vi "Fractal.vi"() -> ()   [LabVIEW 2012]
uses:
  typedefs/t_LuaVIEW Reference.ctl
  subvis/private/LuaVIEW Pull (number).vi
  subvis/private/LuaVIEW Pull (U32).vi
  subvis/private/LuaVIEW Push (number).vi
panel:
  out "picture":picture
  # "This example uses a Lua-driven state machine to draw a fractal. Recursive and numerical algorithms\nare difficult to implement with elegance in LabVIEW, Lua by default has no support for graphics.\nTherefore the recursion and calculations are done with Lua, and the drawing with LabVIEW."
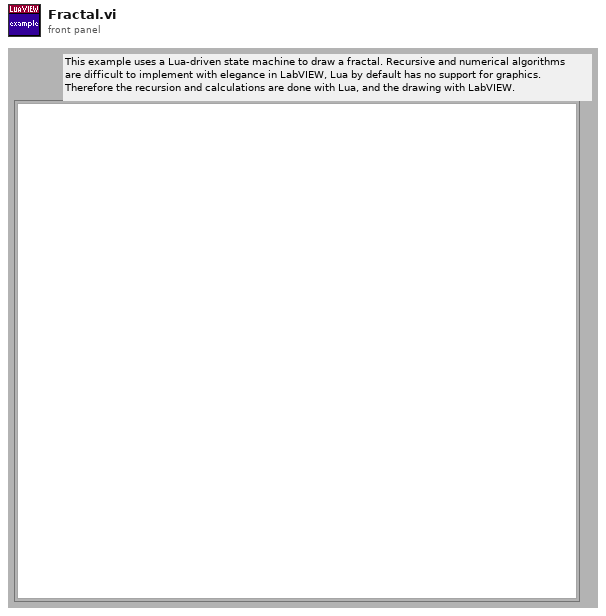
[diagram p1: front panel]
types:
  T1 = enum32{"execute", "initialize", "clear()", "line(num:x1,num:y1,num:x2,num:y2,U32:colour)", "num:width,num:height = dimensions()", "cleanup"}
  T2 = typedef "t_LuaVIEW Reference.ctl" = refnum<k1>
  T3 = typedef "LVBoundsTypeDef.ctl" = cluster{"Width":u32, "Height":u32}
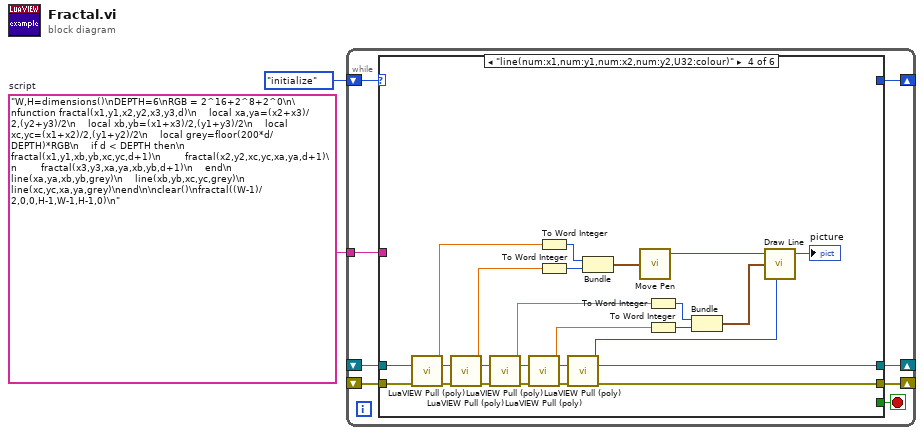
[diagram p0: block diagram]
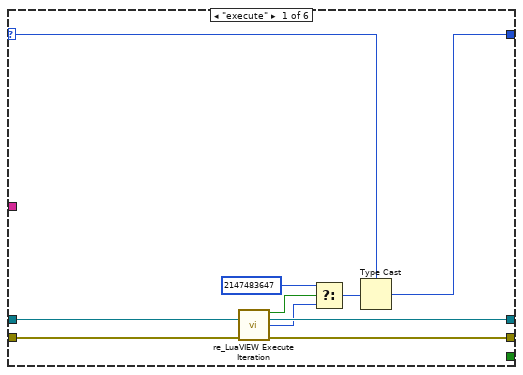
[diagram p2: hidden frame]
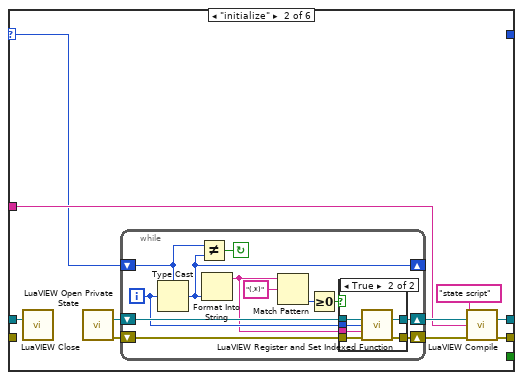
[diagram p3: hidden frame]
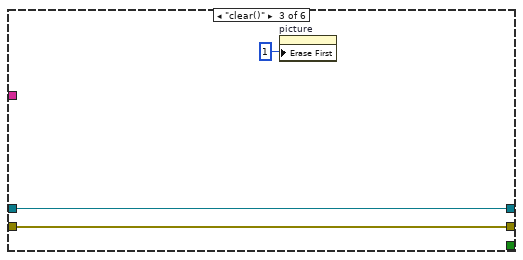
[diagram p5: hidden frame]
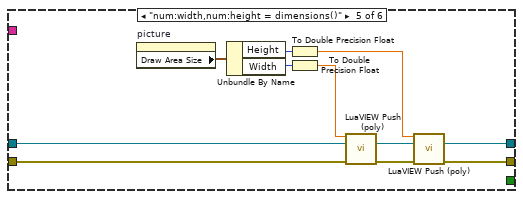
[diagram p6: hidden frame]
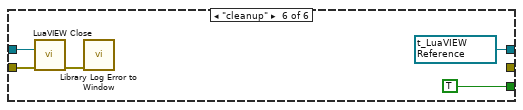
[diagram p7: hidden frame]
diagram:
  w1 = "W,H=dimensions()\nDEPTH=6\nRGB = 2^16+2^8+2^0\n\nfunction fractal(x1,y1,x2,y2,x3,y3,d)\n    local xa,ya=(x2+x3)/2,(y2+y3)/2\n    local xb,yb=(x1+x3)/2,(y1+y3)/2\n    local xc,yc=(x1+x2)/2,(y1+y2)/2\n    local grey=floor(200*d/DEPTH)*RGB\n    if d < DEPTH then\n        fractal(x1,y1,xb,yb,xc,yc,d+1)\n        fractal(x2,y2,xc,yc,xa,ya,d+1)\n        fractal(x3,y3,xa,ya,xb,yb,d+1)\n    end\n    line(xa,ya,xb,yb,grey)\n    line(xb,yb,xc,yc,grey)\n    line(xc,yc,xa,ya,grey)\nend\n\nclear()\nfractal((W-1)/2,0,0,H-1,W-1,H-1,0)\n"  # script
  n1 = while {
    shift-right: [w8] -> _
    shift-left: T1."initialize" -> [w10]
    shift-right: [w6] -> _
    shift-left: _ -> [w7]
    shift-right: [w5] -> _
    shift-left: _ -> [w4]
    tunnel: w1 -> [w3]
    stop <- w9 stop-if-true
    n2 = case shown="\"line(num:x1,num:y1,num:x2,num:y2,U32:colour)\"" w10 {
      selector: w10 -> [w13 w22 _ _ _ _]
      tunnel: [_ _ _ _ _ TRUE] -> w9
      tunnel: [w11 _ _ _ _ _] -> w8
      tunnel: w7 -> [w20 w30 w53 w69 w86 w94]
      tunnel: [w17 w25 w53 w60 w82 w93] -> w6
      tunnel: [w18 w21 w51 w55 w81 _] -> w5
      tunnel: w4 -> [w19 _ w51 w70 w85 w91]
      tunnel: w3 -> [_ w23 _ _ _ _]
      frame "execute" {
        n3 = call "re_LuaVIEW Execute Iteration.vi"("LuaVIEW reference in"=w20, "init or indexed function error"=w19) -> ("last?"=w15:bool, "LuaVIEW reference out"=w17:T2, "function index"=w16:i32, "final error"=w18:errorcluster)  [unwired: 10 in]
        n4 = Select(t=2147483647, s=w15, f=w16) -> (s? t:f=w12:i32)
        n5 = Type Cast(type=w13, x=w12) -> (*(type *) &x=w11:T1)
      }
      frame "initialize" {
        n6 = call "LuaVIEW Close.vi"("LuaVIEW reference"=w30) -> ()  [unwired: 14 in, 1 out]
        n7 = call "LuaVIEW Open Private State.vi"() -> ("LuaVIEW reference"=w28:T2, "error out"=w29:errorcluster)  [unwired: 14 in]
        n8 = while {
          shift-right: [w36] -> w27
          shift-left: w29 -> [w39]
          shift-right: [w37] -> w26
          shift-left: w28 -> [w38]
          shift-right: [w31] -> _
          shift-left: w22 -> [w32]
          i -> [w35]
          stop <- w42 continue-if-true
          n9 = Type Cast(type=w32, x=w35) -> (*(type *) &x=w31:T1)
          n10 = Not Equal?(x=w32, y=w31) -> (x != y?=w42:bool)
          n11 = Format Into String(w31) -> (resulting string=w33:string)  [unwired: 3 in, 1 out]
          n12 = Match Pattern(string=w33, regular expression="(.*)") -> (offset past match=w40:i32)  [unwired: 1 in, 3 out]
          n13 = Greater Or Equal To 0?(x=w40) -> (x >= 0?=w34:bool)
          n14 = case shown="True" w34 {
            tunnel: w38 -> [w44 w47]
            tunnel: w35 -> [_ w48]
            tunnel: w33 -> [_ w45]
            tunnel: [w43 w50] -> w36
            tunnel: [w44 w49] -> w37
            tunnel: w39 -> [w43 w46]
            frame False {
            }
            frame True {
              n15 = call "LuaVIEW Register and Set Indexed Function.vi"("LuaVIEW reference in"=w47, "index"=w48, "synopsis"=w45, "error in (no error)"=w46) -> ("LuaVIEW reference out"=w49:T2, "error out"=w50:errorcluster)  [unwired: 10 in]
            }
          }
        }
        n16 = call "LuaVIEW Compile.vi"("script name"="state script", "LuaVIEW reference in"=w26, "script"=w23, "error in (no error)"=w27) -> ("LuaVIEW reference out"=w25:T2, "error out"=w21:errorcluster)  [unwired: 10 in]
      }
      frame "clear()" {
        n17 = property on="picture" class="Pict"("Erase First"=u8 1) -> ()  [unwired: 2 in, 2 out]
      }
      frame "line(num:x1,num:y1,num:x2,num:y2,U32:colour)" {
        n18 = call-poly "LuaVIEW Pull (poly).vi"("LuaVIEW reference in"=w69, "error in (no error)"=w70) -> ("number"=w59:dbl, "LuaVIEW reference out"=w68:T2, "error out"=w67:errorcluster)  [unwired: 11 in]
        n19 = call-poly "LuaVIEW Pull (poly).vi"("LuaVIEW reference in"=w68, "error in (no error)"=w67) -> ("number"=w58:dbl, "LuaVIEW reference out"=w66:T2, "error out"=w65:errorcluster)  [unwired: 11 in]
        n20 = call-poly "LuaVIEW Pull (poly).vi"("LuaVIEW reference in"=w66, "error in (no error)"=w65) -> ("number"=w57:dbl, "LuaVIEW reference out"=w64:T2, "error out"=w63:errorcluster)  [unwired: 11 in]
        n21 = call-poly "LuaVIEW Pull (poly).vi"("LuaVIEW reference in"=w64, "error in (no error)"=w63) -> ("number"=w56:dbl, "LuaVIEW reference out"=w62:T2, "error out"=w61:errorcluster)  [unwired: 11 in]
        n22 = To Word Integer(number=w59) -> (16bit integer=w77:i16)
        n23 = To Word Integer(number=w58) -> (16bit integer=w76:i16)
        n24 = call-poly "LuaVIEW Pull (poly).vi"("LuaVIEW reference in"=w62, "error in (no error)"=w61) -> ("U32"=w54:u32, "LuaVIEW reference out"=w60:T2, "error out"=w55:errorcluster)  [unwired: 11 in]
        n25 = Bundle(w77, w76) -> (w75:cluster{i16, i16})  [unwired: 1 in]
        n26 = call <vilib>:"Move Pen.vi"("new position"=w75) -> ("new picture"=w78:picture)  [unwired: 4 in]
        n27 = To Word Integer(number=w57) -> (16bit integer=w73:i16)
        n28 = To Word Integer(number=w56) -> (16bit integer=w74:i16)
        n29 = Bundle(w73, w74) -> (w72:cluster{i16, i16})  [unwired: 1 in]
        n30 = call <vilib>:"Draw Line.vi"("picture"=w78, "end point"=w72, "color(black)"=w54) -> ("new picture"=→"picture":picture)  [unwired: 6 in]
      }
      frame "num:width,num:height = dimensions()" {
        n31 = property on="picture" class="Pict"() -> ("Draw Area Size"=w89:T3)  [unwired: 2 in, 2 out]
        n32 = Unbundle By Name(w89) -> ("Height"=w88:u32, "Width"=w87:u32)
        n33 = To Double Precision Float(number=w88) -> (double precision float=w79:dbl)
        n34 = To Double Precision Float(number=w87) -> (double precision float=w80:dbl)
        n35 = call-poly "LuaVIEW Push (poly).vi"("number"=w80, "LuaVIEW reference in"=w86, "error in (no error)"=w85) -> ("LuaVIEW reference out"=w83:T2, "error out"=w84:errorcluster)  [unwired: 11 in]
        n36 = call-poly "LuaVIEW Push (poly).vi"("number"=w79, "LuaVIEW reference in"=w83, "error in (no error)"=w84) -> ("LuaVIEW reference out"=w82:T2, "error out"=w81:errorcluster)  [unwired: 11 in]
      }
      frame "cleanup" {
        w93 = T2 refnum items=["LuaVIEW"] ("LuaVIEW reference")
        n37 = call "LuaVIEW Close.vi"("LuaVIEW reference"=w94, "error in (no error)"=w91) -> ("dup error"=w90:errorcluster)  [unwired: 13 in]
        n38 = call "Library Log Error to Window.vi"("error in (no error)"=w90) -> ()  [unwired: 13 in, 2 out]
      }
    }
  }
